vi "AbortGeneration.vi"(8 "error in (no error)":errorcluster, 11 "ClassIn":refnum<class "Keysight335XX.lvclass">) -> (0 "error out":errorcluster, 3 "ClassOut":refnum<class "Keysight335XX.lvclass">)   [LabVIEW 2014, in "FGenPlugins.lvlib" / "Keysight335XX.lvclass"]
uses:
  Keysight335XX.lvclass
  <instrlib>/Agilent 3352X Series/Agilent 3352X Series.lvlib
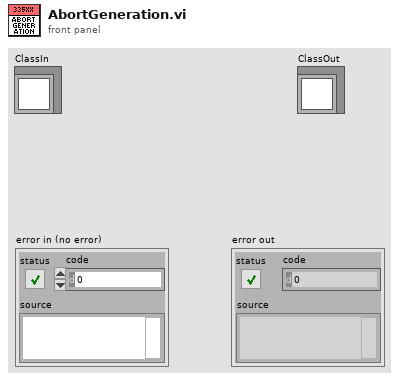
[diagram p1: front panel]
types:
  T1 = typedef "FGenPlugins.lvlib/NISTFGenPluginsBase.lvclass/ChannelParamElement.ctl" = cluster{"sName":string, "eOperateMode":u16, "bEnabled":bool, "eOutputMode":u16, "iIndex":i32, "iNameBufferSize":i32, "fGain":dbl}
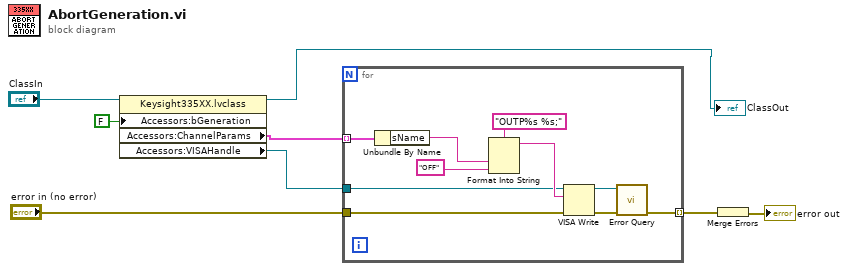
[diagram p0: block diagram]
diagram:
  n1 = property class="Keysight335XX.lvclass"(reference="ClassIn", "Accessors:bGeneration"=FALSE ("bGeneration")) -> (reference out=→"ClassOut":refnum<class "Keysight335XX.lvclass">, "Accessors:ChannelParams"=w7:T1[], "Accessors:VISAHandle"=w6:refnum<visa-resource-name>)  [unwired: 1 in, 1 out]
  n2 = for {
    tunnel: w7 -> [w18] mode=indexing
    tunnel: w6 -> [w13]
    tunnel: "error in (no error)" -> [w12]
    tunnel: [w10] -> w3 mode=indexing
    n3 = Unbundle By Name(w18) -> ("sName"=w14:string)
    n4 = Format Into String(format string="OUTP%s %s;", w14, "OFF") -> (resulting string=w16:string)  [unwired: 2 in, 1 out]
    n5 = VISA Write(VISA resource name=w13, write buffer=w16, error in (no error)=w12) -> (VISA resource name out=w17:refnum<visa-resource-name>, error out=w11:errorcluster)  [unwired: 1 out]
    n6 = call <instrlib>:"Error Query.vi"("error in (no error)"=w11, "VISA resource name"=w17) -> ("error out"=w10:errorcluster)  [unwired: 9 out]
  }
  n7 = Merge Errors(w3) -> (→"error out":errorcluster)
